vi "SEC code V3.0.1.121.vi"() -> ()   [LabVIEW 2020]
uses:
  SEC code V3.0.1/Drivers and Aux files/IVIUM/IVIUM_remdriver.lvlib
  SEC code V3.0.1/Drivers and Aux files/State.ctl
  SEC code V3.0.1/Drivers and Aux files/SECenumctl.ctl
  SEC code V3.0.1/Drivers and Aux files/OSSPEC.ctl
panel:
  out "?":T1(graph)
  in  "Tab Control 2":T2(tab)
  in  "V 1 time (s)":dbl
  in  "V off time":dbl
  in  "Sampling time (s)":dbl
  in  "V 2 time (s)":dbl
  in  "Run OSPSEC":bool
  out "System potential":dbl
  in  "V1 (V)":dbl
  in  "V2 (V)":dbl
  in  "Reverse Scan\ndirection":bool
  in  "File Name":string="test-1"
  in  "Path":path=path "C:/Users/LocalAdmin/Desktop"
  out "cell on":bool
  in  "Tab Control":T3(tab)
  out "?":T1(graph)
  out "?":T1(graph)
  out "?":cluster{dbl[], dbl[]}(graph)
  out "I_overload":bool
  out "Aninput1_overload":bool
  out "E_overload":bool
  out "cell-off button pressed":bool
  in  "Default\nCurrent range":T4(ring)=enum."100 uA"
  in  "Default Filter":T5(ring)=enum."10 kHz"
  out "Device serial number":string
  in  "Set Stability":T6(ring)=enum."Standard"
  out "Number of Spectrometers":i32
  out "Values to re-intialise to at end\nof the measument":T7
  in  "Equilibration \ntime (s)":u32=5
  in  "Wait before \nspectrum (s)":dbl=0.1
  in  "Inetegration Time (us)":i32=10000
  in  "Continuous \nStrobe Delay (us)":i32
  in  "Increment (V)":dbl=0.01
  in  "Stop potential (V)":dbl=0.4
  in  "Default Potential (V)":dbl=-0.4
  in  "Start potential (V)":dbl=-0.4
  in  "Exit and disconnect":bool
  out "current":dbl caption="Current (A)" format="%_4g"
  out "V (during measurment)":dbl
  out "Potentiostat Status":string
  in  "(update and read)":bool
  # "OSPSEC control"
  # "Program control"
  # "Spectrometer control"
  # "Potentiostat Status"
  # "SEC control"
  # "Cell on?"
  # "I overload overload"
  # "off button pressed"
  # "Aninput1 overload"
  # "E overload"
  # "OSPEC loop exit"
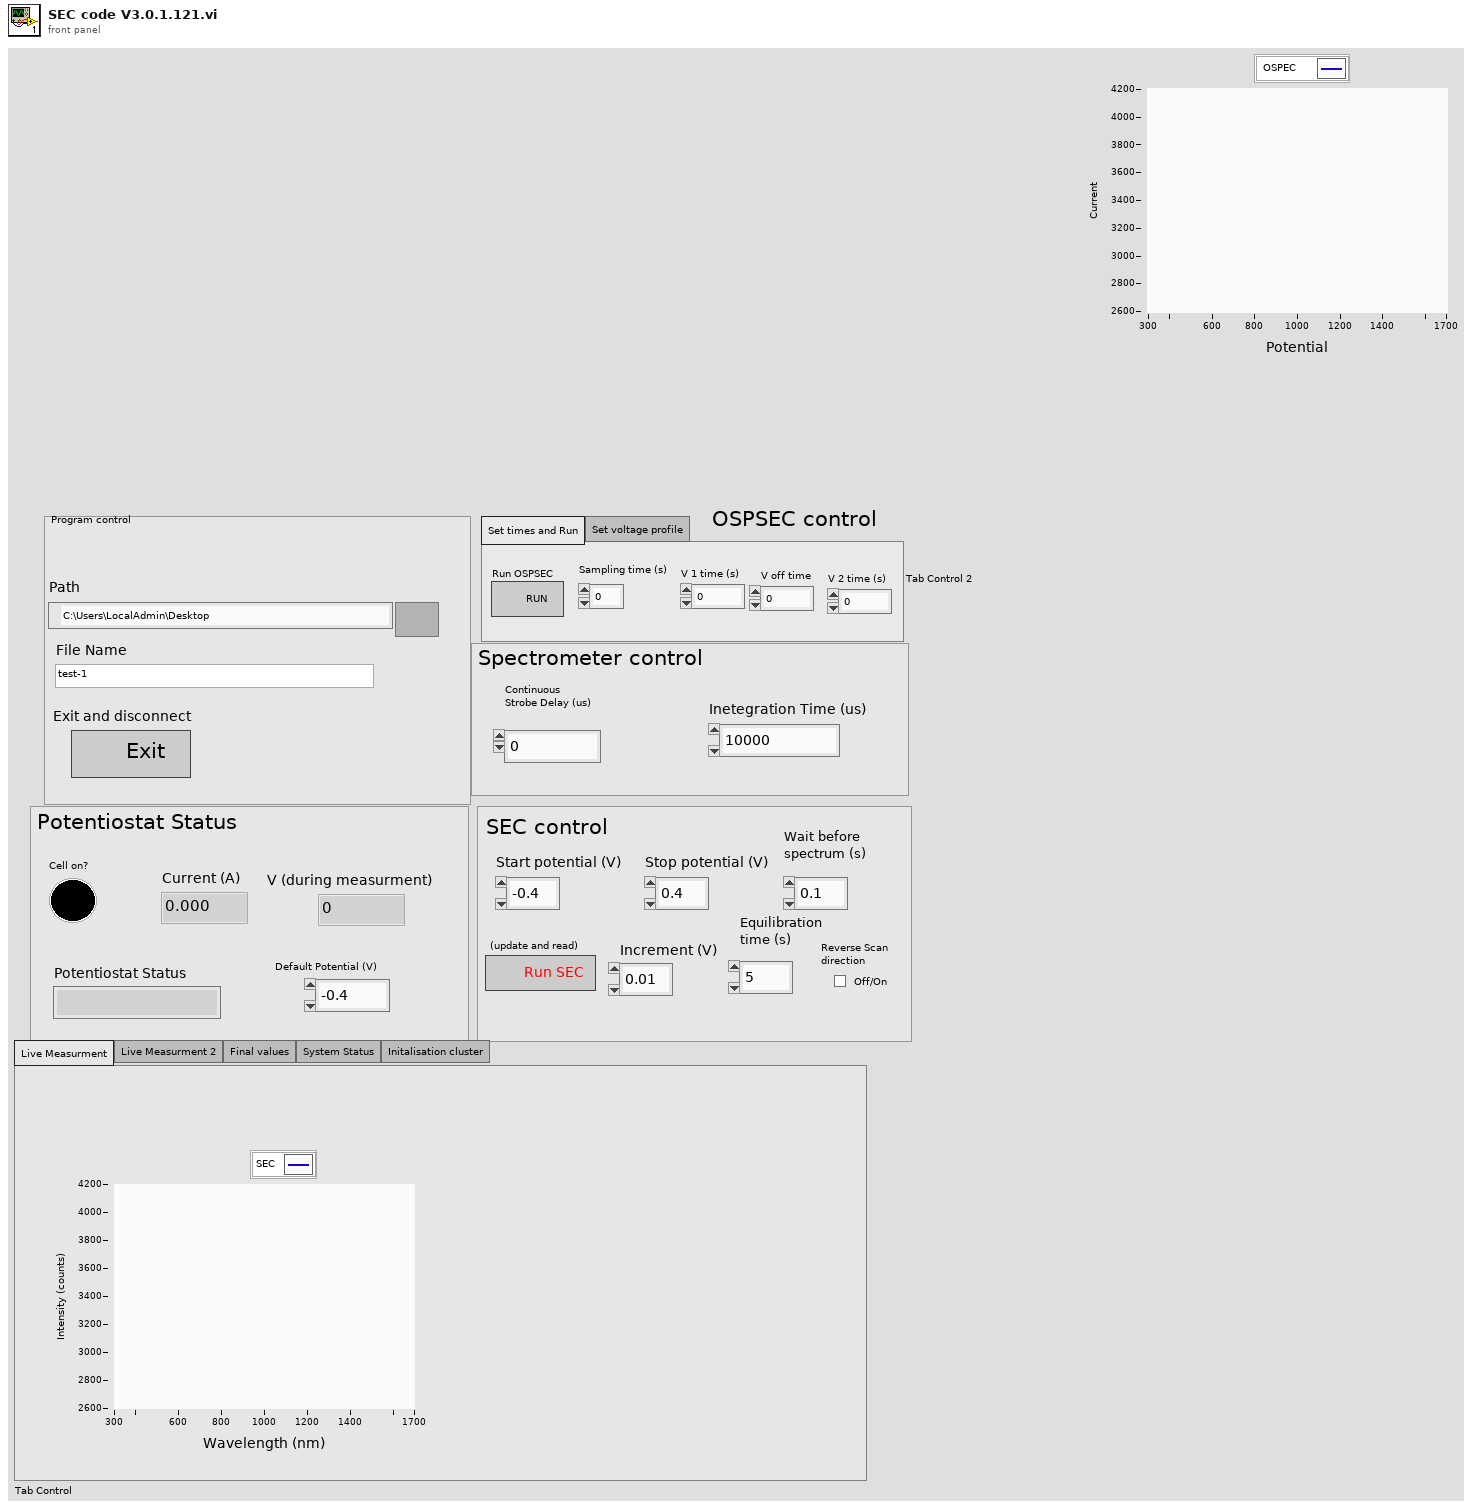
[diagram p1: front panel]
types:
  T1 = cluster{"WL Values":dbl[], "Spectrum Values":dbl[]}
  T2 = enum32{"Set times and Run", "Set voltage profile"}
  T3 = enum32{"Live Measurment", "Live Measurment 2", "Final values", "System Status", "Initalisation cluster"}
  T4 = enum16{"10 A", "1 A", "100 mA", "10 mA", "1 mA", "100 uA", "10 uA", "1 uA", "100 nA", "10 nA", "1 nA", "100 pA", "10 pA", "1 pA"}
  T5 = enum16{"1 MHz", "100 kHz", "10 kHz", "1 kHz", "10 Hz"}
  T6 = enum16{"High Speed", "Standard", "High Stability"}
  T7 = cluster{"Currents":dbl[], "Potentials":dbl[], "Device Status":string, "Device serial no":string, "Current":dbl, "Default \nPotential":dbl, "I overload":bool, "Cell On":bool, "E overload":bool, "Aninput1 overload":bool, "Cell off button pressed":bool, "Start potential":dbl, "Stop potential":dbl, "Increment":dbl, "SEC":dbl[], "Path":path, "File name":string}
  T8 = cluster{"Current array":dbl[], "Potential array":dbl[], "Status":string, "Serial No":string, "Current":dbl, "Default\n potential":dbl, "I overload":bool, "Cell on":bool, "E overload":bool, "Cell of button pressed":bool, "Aninput1 overload":bool, "Stop \npotential":dbl, "Start \npotential":dbl, "Increment":dbl, "Spectrum":dbl[][], "Path":path, "File Name":string, "Sample rate":dbl, "V2 time":dbl, "V off time":dbl, "V 2":dbl, "V 1":dbl, "V1 time":dbl, "Time array":dbl[], "Integration time":i32, "Continous strobe delay":i32, "Time elapsed ":i32, "Start time":i32}
  T9 = typedef "State.ctl" = enum16{"Initialize", "Wait for Event", "Run SEC", "Run OSPEC", "Output data and process", "Exit"}
  T10 = typedef "SECenumctl.ctl" = enum16{"Read spectrum", "Apply potential", "Wait"}
  T11 = typedef "OSSPEC.ctl" = enum16{"Read Potential and spectrum", "Read current and spectrum", "Reinitialise Cell", "Apply V1", "Apply V2"}
  T12 = typedef "Rendezvous RefNum" = refnum<k1>
  T13 = cluster{"Spectrum Values":dbl[], "WL Values":dbl[]}
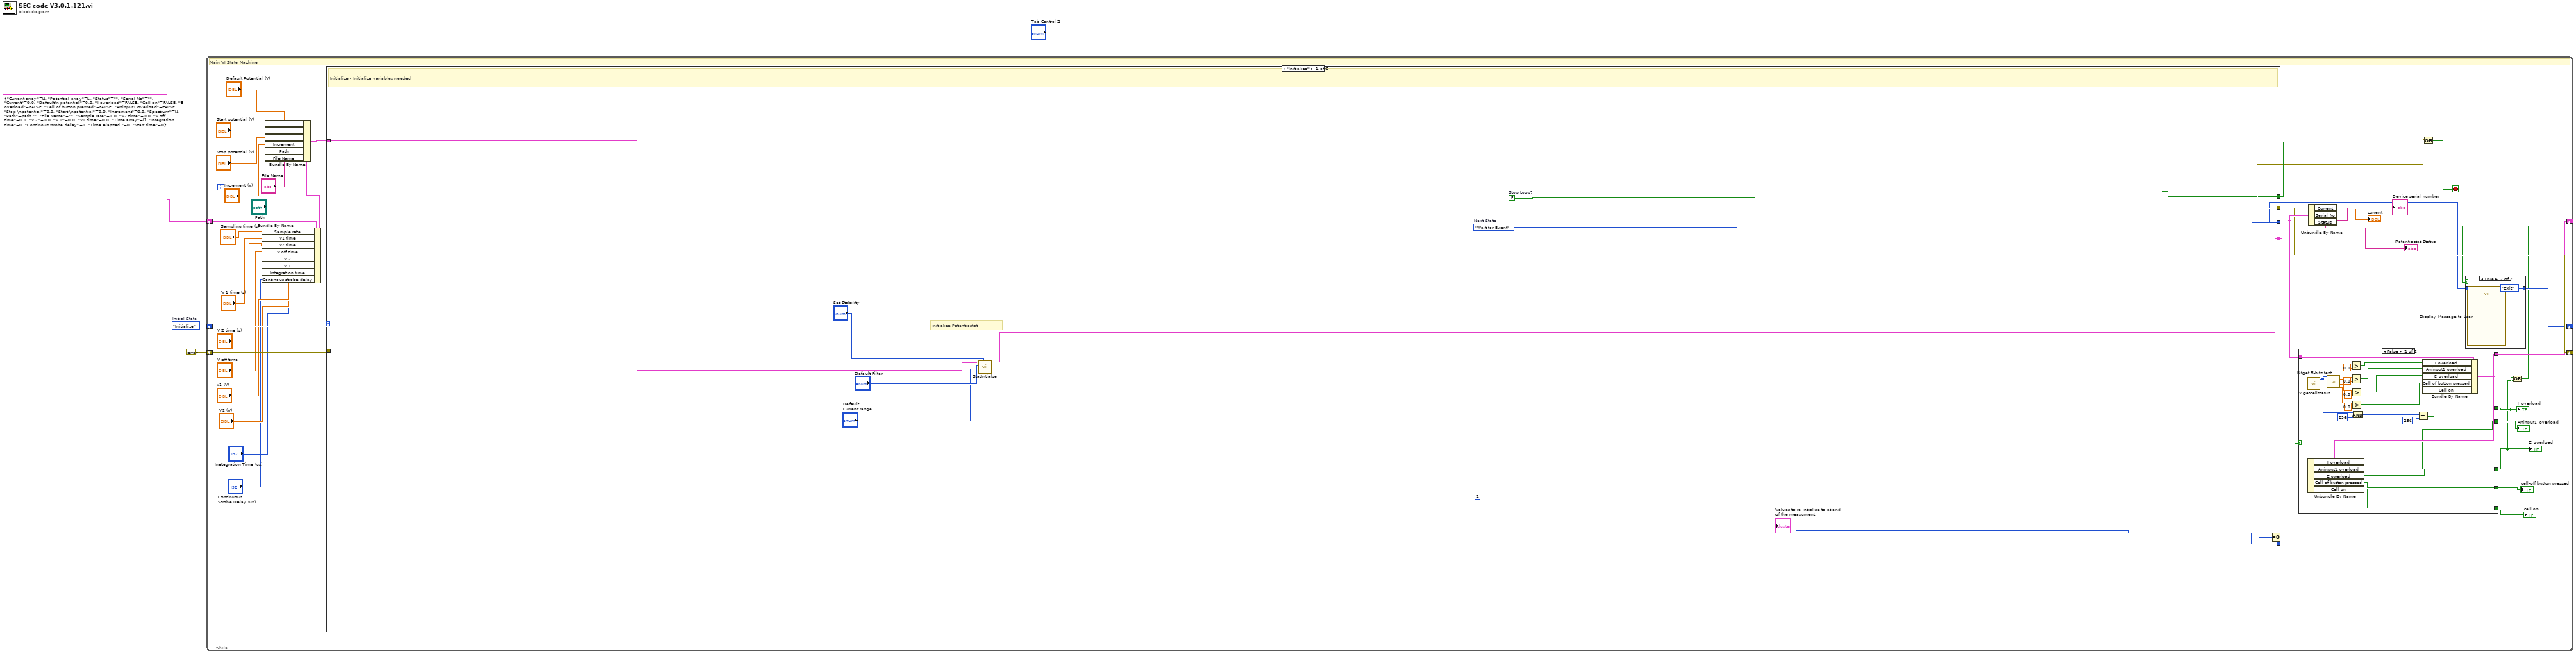
[diagram p0: block diagram]
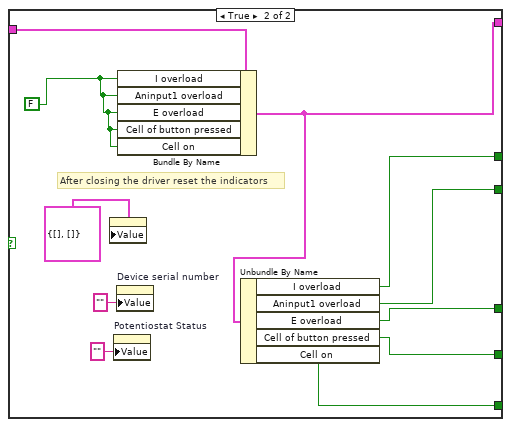
[diagram p3: hidden frame]
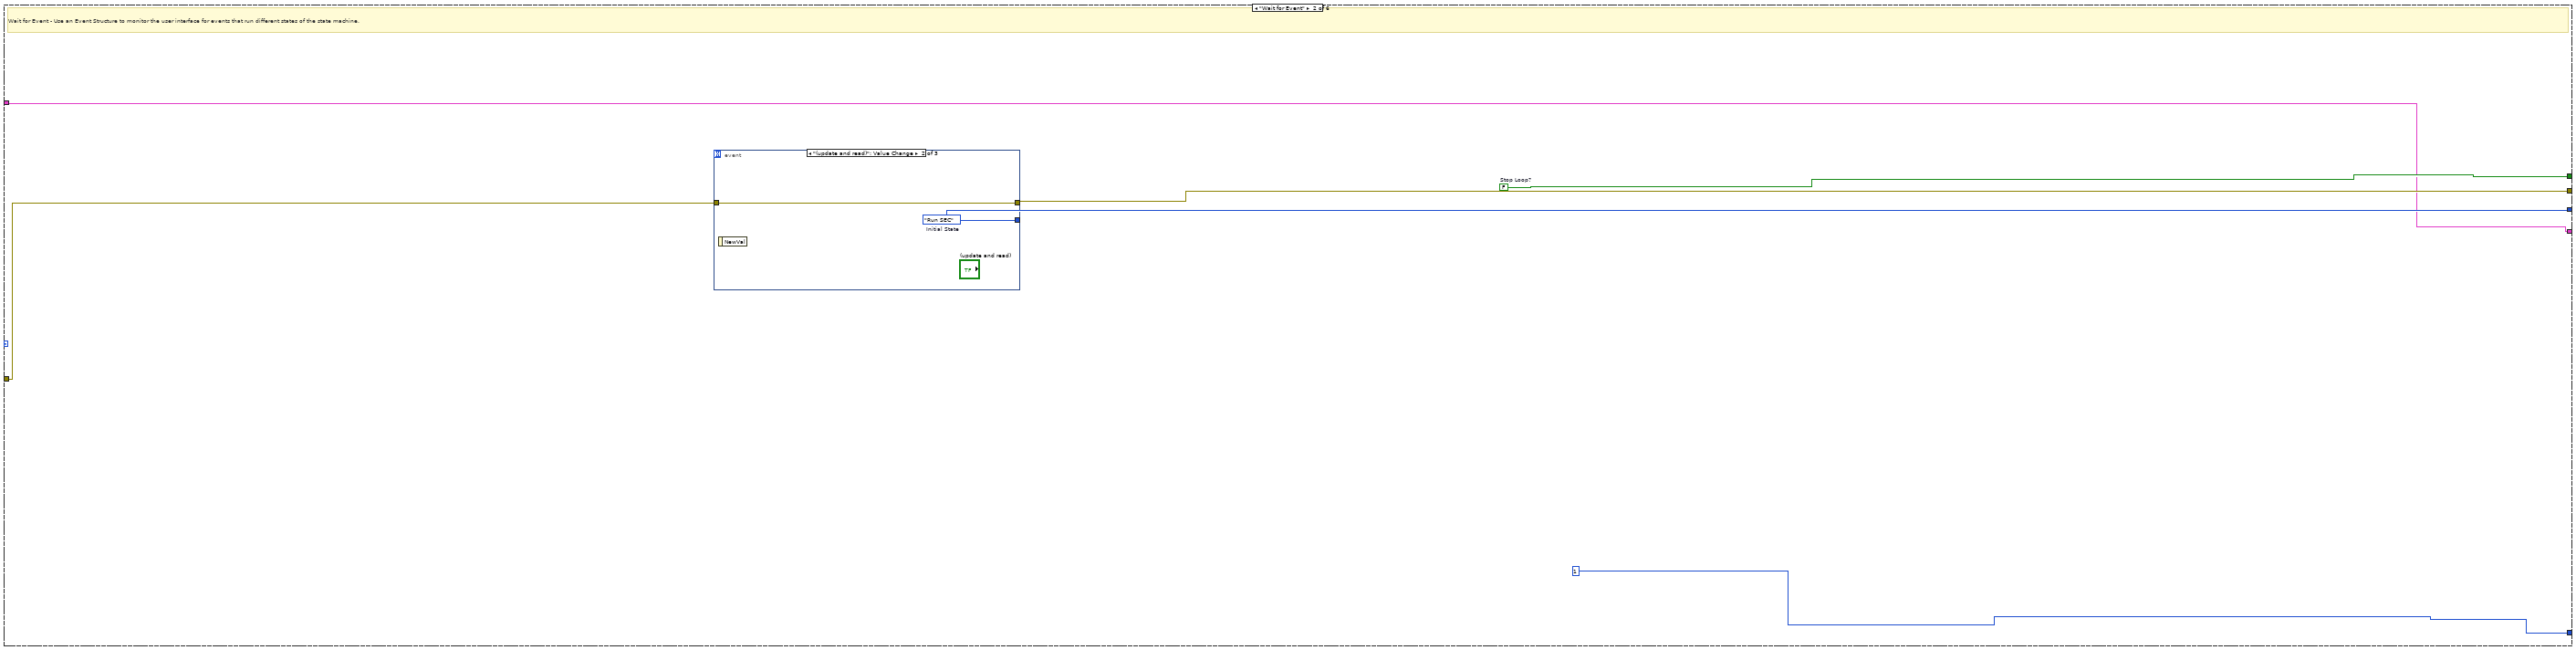
[diagram p4: hidden frame]
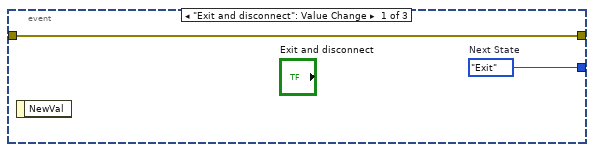
[diagram p5: hidden frame]
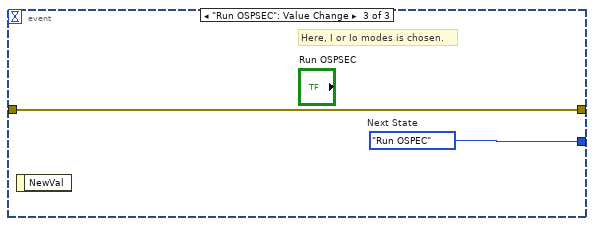
[diagram p6: hidden frame]
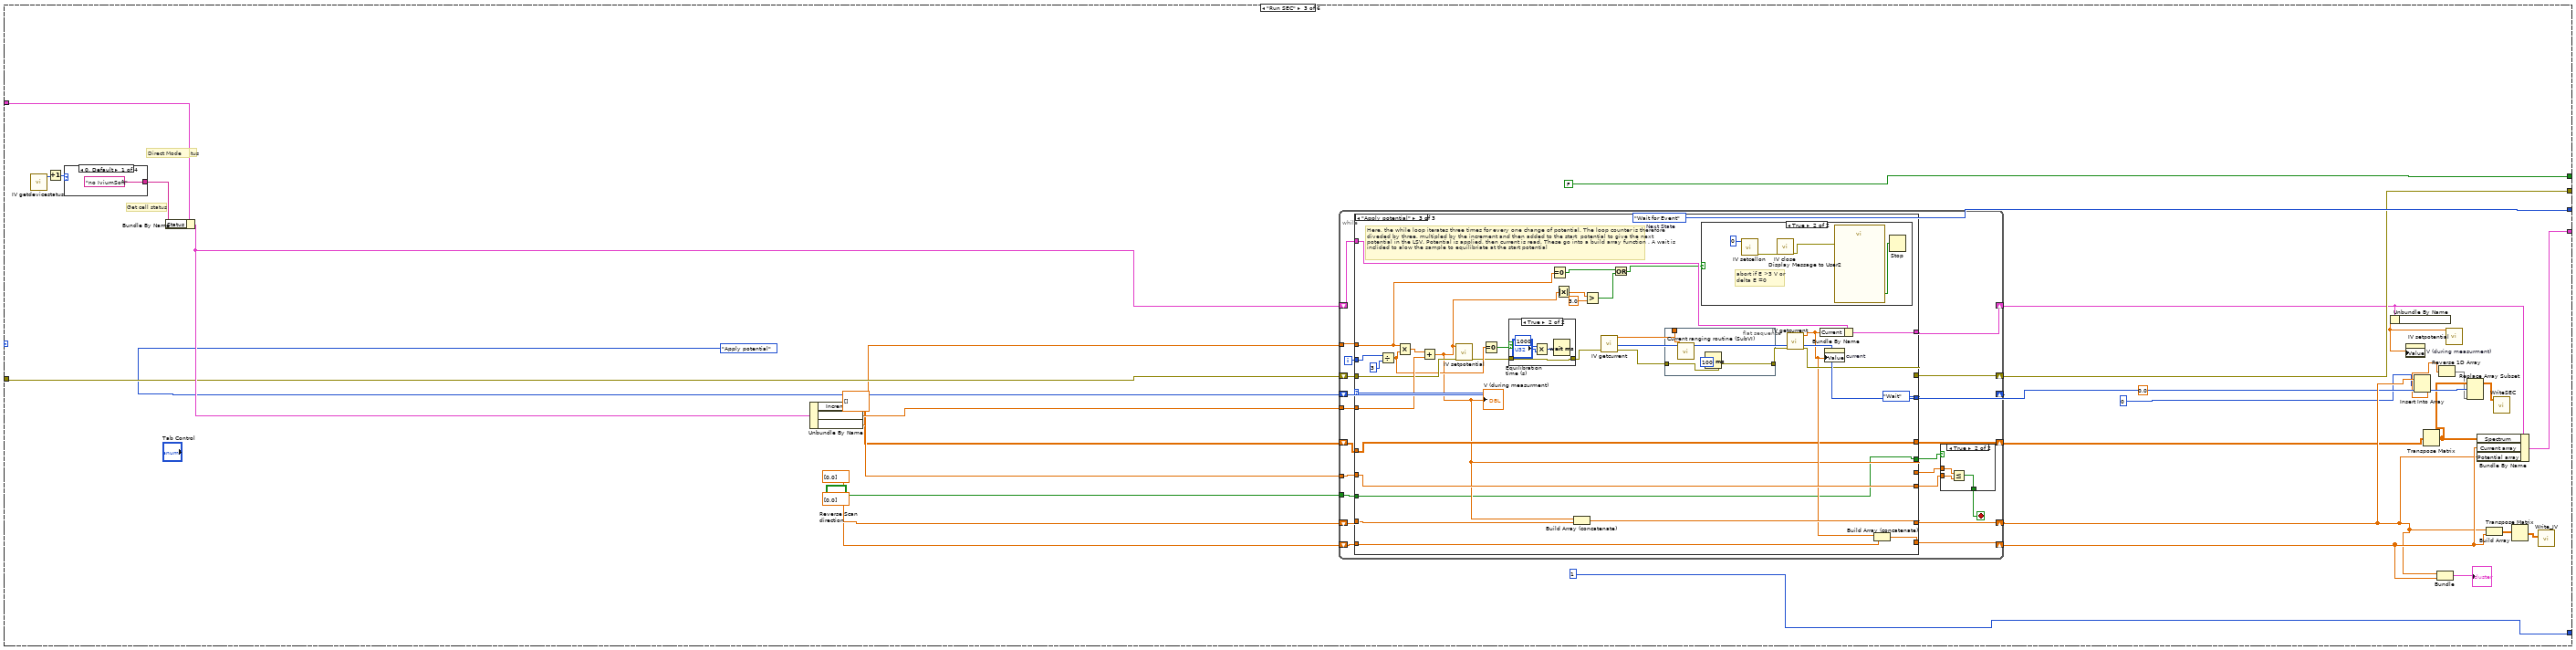
[diagram p7: hidden frame]
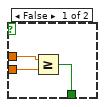
[diagram p8: hidden frame]
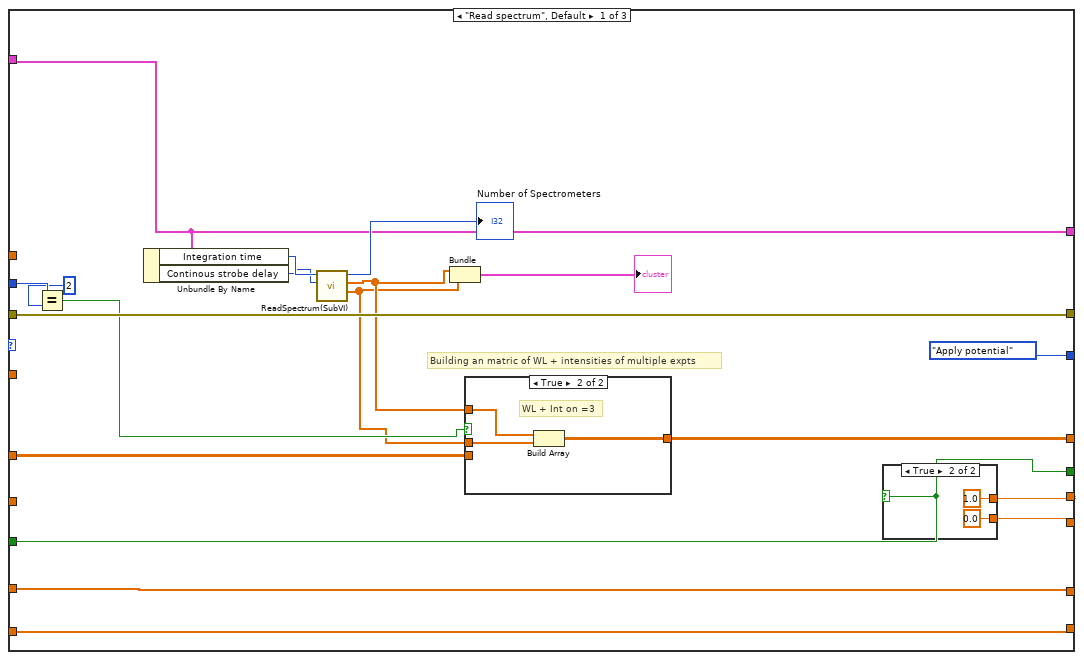
[diagram p9: hidden frame]
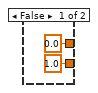
[diagram p10: hidden frame]
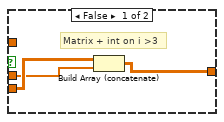
[diagram p11: hidden frame]
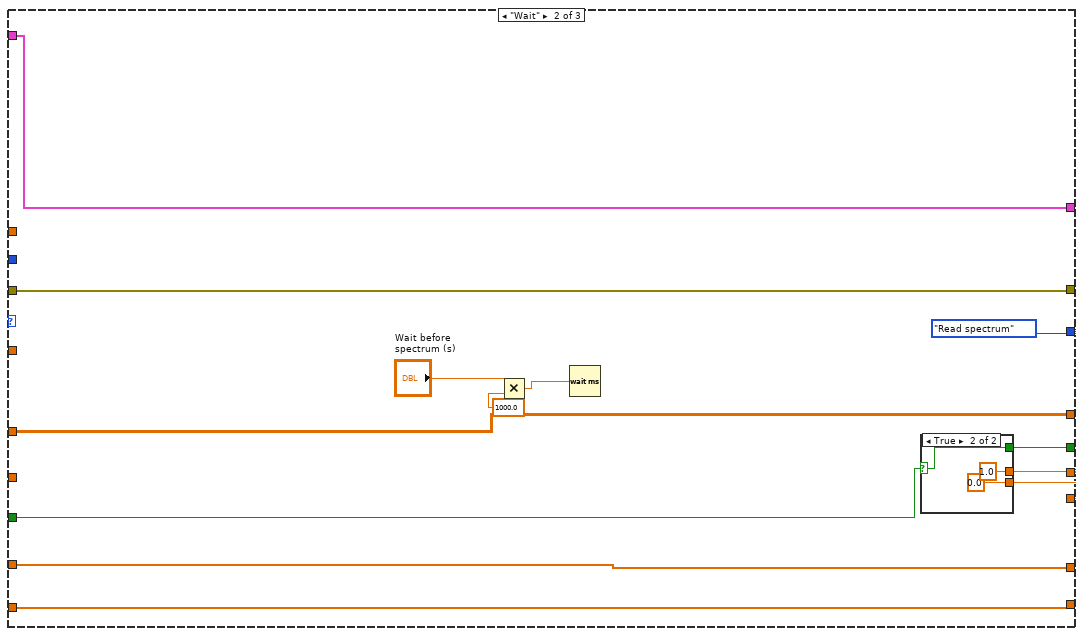
[diagram p12: hidden frame]
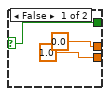
[diagram p13: hidden frame]
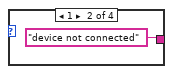
[diagram p16: hidden frame]
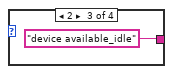
[diagram p17: hidden frame]
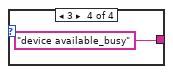
[diagram p18: hidden frame]
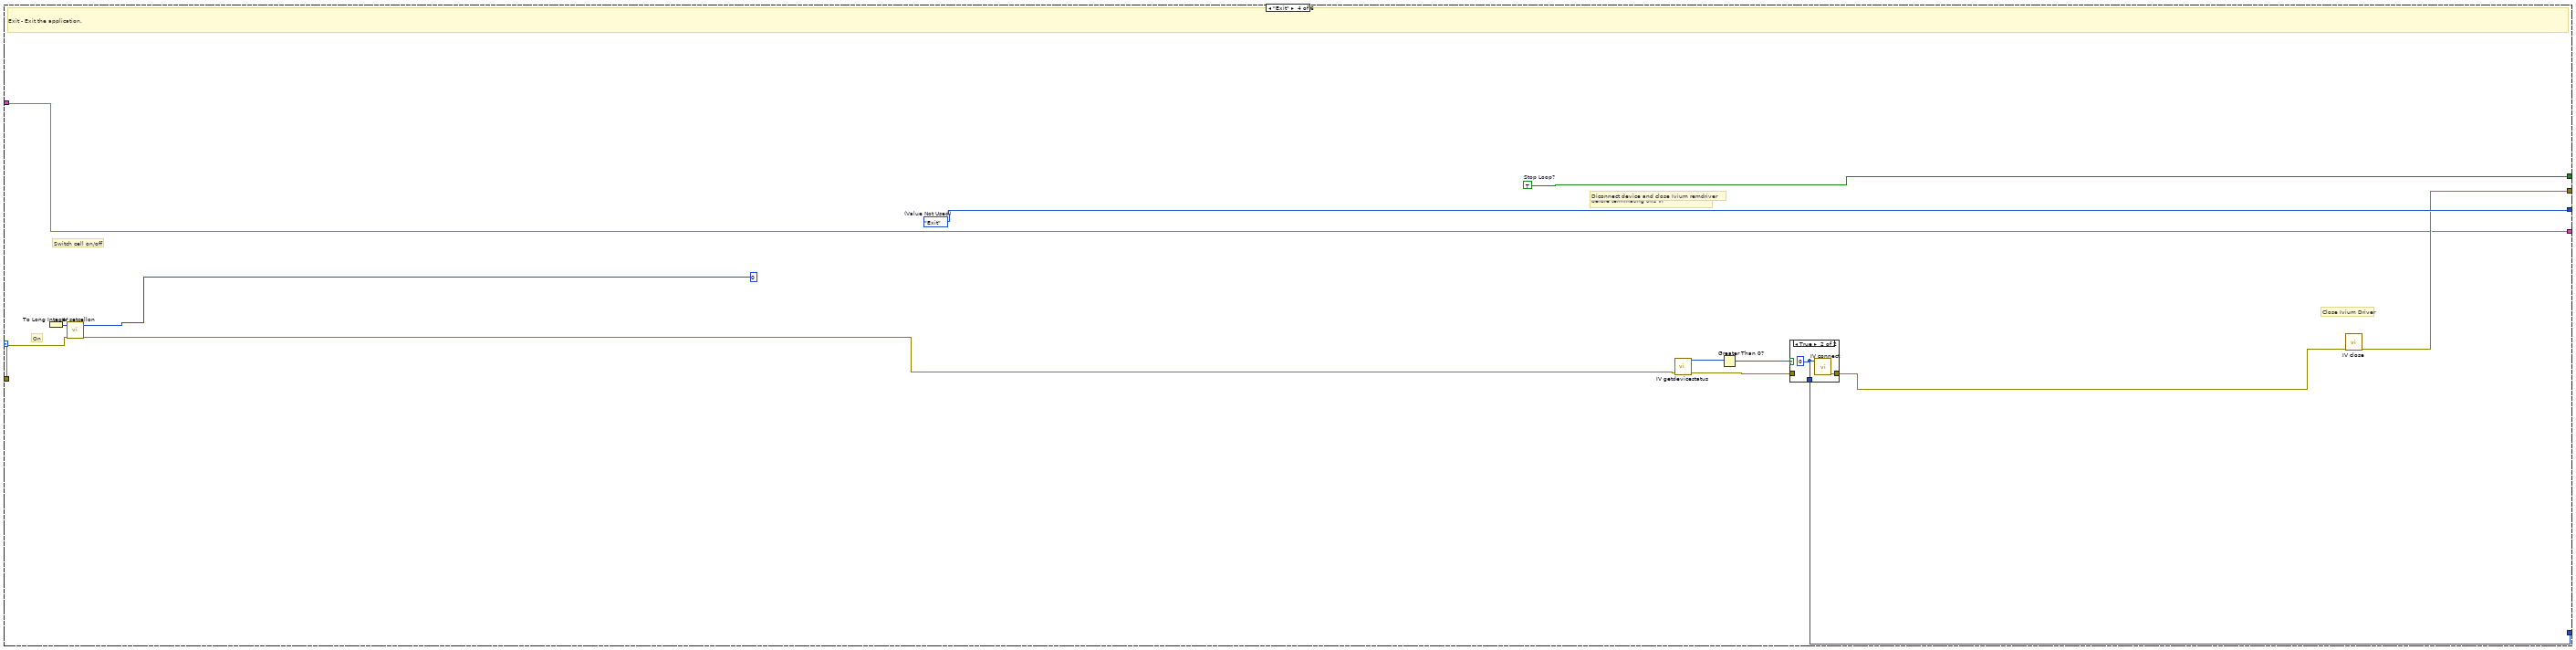
[diagram p19: hidden frame]
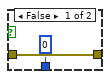
[diagram p20: hidden frame]
diagram:
  w3 = State."Initialize"  # Initial State
  n1 = while {
    shift-right: [w20] -> _
    shift-left: w3 -> [w40]
    shift-right: [w25] -> _
    shift-left: T8 {"Current array"=[], "Potential array"=[], "Status"="", "Serial No"="", "Current"=0.0, "Default\n potential"=0.0, "I overload"=FALSE, "Cell on"=FALSE, "E overload"=FALSE, "Cell of button pressed"=FALSE, "Aninput1 overload"=FALSE, "Stop \npotential"=0.0, "Start \npotential"=0.0, "Increment"=0.0, "Spectrum"=[], "Path"=path "", "File Name"="", "Sample rate"=0.0, "V2 time"=0.0, "V off time"=0.0, "V 2"=0.0, "V 1"=0.0, "V1 time"=0.0, "Time array"=[], "Integration time"=0, "Continous strobe delay"=0, "Time elapsed "=0, "Start time"=0} -> [w13]
    shift-right: [w26] -> _
    shift-left: errorcluster {"status"=FALSE, "code"=0, "source"=""} ("error constant") -> [w39]
    stop <- w37 stop-if-true
    # "Main VI State Machine"
    n2 = Bundle By Name(cluster=w13, "Sample rate"="Sampling time (s)", "V1 time"="V 1 time (s)", "V2 time"="V 2 time (s)", "V off time"="V off time", "V 2"="V1 (V)", "V 1"="V2 (V)", "Integration time"="Inetegration Time (us)", "Continous strobe delay"="Continuous \nStrobe Delay (us)") -> (w4:T8)
    n3 = Bundle By Name(cluster=w4, "Default\n potential"="Default Potential (V)", "Start \npotential"="Start potential (V)", "Stop \npotential"="Stop potential (V)", "Increment"="Increment (V)", "Path"="Path", "File Name"="File Name") -> (w22:T8)
    n4 = case shown="\"Initialize\"" w40 {
      tunnel: [w84 w91 w129 w266 State."Wait for Event" ("f") State."Wait for Event" ("f")] -> w16
      tunnel: [w83 w88 FALSE ("Stop Loop?") w254 FALSE ("Stop Loop?") _] -> w38
      tunnel: w22 -> [w79 w86 w114 w255 w277 w676]
      tunnel: [w78 w86 w104 w255 w272 w676] -> w33
      tunnel: w39 -> [_ w90 w123 w258 w275 w679]
      tunnel: [_ w89 w122 w261 w273 w679] -> w26
      tunnel: [1 ("devconnect") 1 ("devconnect") 1 ("devconnect") w256 1 ("devconnect") 1 ("devconnect")] -> w21
      frame "Initialize" {
        w83 = FALSE  # Stop Loop?
        w84 = State."Wait for Event"  # Next State
        # "initialize Potentiostat"
        # "Initialize - Initialize variables needed"
        n5 = call "StatIntialse.vi"("Set Stability"="Set Stability", "Default\nCurrent range"="Default\nCurrent range", "Default\n Filter"="Default Filter", "Cluster in"=w79) -> ("Cluster out"=w78:T8)  [unwired: 6 in, 1 out]
      }
      frame "Wait for Event" {
        w88 = FALSE  # Stop Loop?
        # "Wait for Event - Use an Event Structure to monitor the user interface for events that run different states of the state machine."
        n6 = event shown="[1] \"(update and read)\": Value Change" {
          selector: _ -> [_ _ _]
          dyn-events: _ -> [_ _ _]
          timeout: _ -> [_ _ _]
          tunnel: [w93 w94 w97] -> w91
          tunnel: w90 -> [w92 w95 w96]
          tunnel: [w92 w95 w96] -> w89
          event "Exit and disconnect": Value Change {
            w93 = State."Exit"  # Next State
            n7 = event-data() -> ()  [unwired: 1 in, 1 out]
          }
          event "(update and read)": Value Change {
            w94 = State."Run SEC"  # Initial State
            n8 = event-data() -> ()  [unwired: 1 in, 1 out]
          }
          event "Run OSPSEC": Value Change {
            w97 = State."Run OSPEC"  # Next State
            # "Here, I or Io modes is chosen."
            n9 = event-data() -> ()  [unwired: 1 in, 1 out]
          }
        }
      }
      frame "Run SEC" {
        w129 = State."Wait for Event"  # Next State
        # "Get cell status"
        # "Get Device Status"
        # "Direct Mode"
        n10 = call "IV getdevicestatus.vi"() -> ("return type"=w127:i32)  [unwired: 10 in, 1 out]
        n11 = Increment(x=w127) -> (x+1=w126:i32)
        n12 = case shown="0, Default" w126 {
          tunnel: ["no IviumSoft" "device not connected" "device available_idle" "device available_busy"] -> w131
          frame 0, Default {
          }
          frame 1 {
          }
          frame 2 {
          }
          frame 3 {
          }
        }
        n13 = Bundle By Name(cluster=w114, "Status"=w131) -> (w125:T8)
        n14 = Unbundle By Name(w125) -> ("Increment"=w120:dbl, "Start \npotential"=w124:dbl, "Stop \npotential"=w115:dbl)
        n15 = while {
          shift-right: [w151] -> w106
          shift-left: w125 -> [w152]
          tunnel: w120 -> [w147]
          tunnel: w124 -> [w146]
          shift-right: [w148] -> w122
          shift-left: w123 -> [w149]
          shift-right: [w140] -> _
          shift-left: SECenumctl."Apply potential" -> [w144]
          shift-right: [w142] -> w111
          shift-left: dbl[] [0.0] -> [w141]
          shift-right: [w137] -> w112
          shift-left: dbl[] [0.0] -> [w138]
          tunnel: w115 -> [w139]
          shift-right: [w136] -> w110
          shift-left: dbl[][] [] -> [w135]
          tunnel: "Reverse Scan\ndirection" -> [w133]
          i -> [w150]
          stop <- w134 stop-if-true
          n16 = case shown="\"Apply potential\"" w144 {
            tunnel: w152 -> [w161 w199 w221]
            tunnel: [w161 w199 w220] -> w151
            tunnel: w150 -> [w170 _ w235]
            tunnel: w149 -> [w171 w195 w232]
            tunnel: [w171 w195 w222] -> w148
            tunnel: w147 -> [_ _ w217]
            tunnel: w146 -> [_ _ w234]
            tunnel: [w177 w198 w214] -> w145
            tunnel: [w176 w197 w227] -> w143
            tunnel: [w175 w196 w225] -> w142
            tunnel: w141 -> [w175 w196 w226]
            tunnel: [SECenumctl."Apply potential" SECenumctl."Read spectrum" SECenumctl."Wait"] -> w140
            tunnel: w139 -> [_ _ w227]
            tunnel: w138 -> [w172 w191 w224]
            tunnel: [w172 w191 w223] -> w137
            tunnel: [w164 w190 w218] -> w136
            tunnel: w135 -> [w163 w190 w218]
            tunnel: w133 -> [w162 w189 w207]
            tunnel: [w162 w188 w207] -> w132
            frame "Read spectrum", Default {
              # "Building an matric of WL + intensities of multiple expts"
              n17 = Equal?(x=w170, y=2) -> (x = y?=w168:bool)
              n18 = Unbundle By Name(w161) -> ("Integration time"=w160:i32, "Continous strobe delay"=w159:i32)
              n19 = call "ReadSpectrum(SubVI).vi"("Continuous \nStrobe Delay"=w159, "Enter the \nInetegration Time"=w160) -> ("Spectrum Values"=w166:dbl[], "WL Values"=w167:dbl[], "Number of Spectrometers"=→"Number of Spectrometers":i32)  [unwired: 7 in]
              n20 = Bundle("WL Values"=w167, "Spectrum Values"=w166) -> (→"?":T1)  [unwired: 1 in]
              n21 = case shown="True" w168 {
                tunnel: w167 -> [_ w187]
                tunnel: w166 -> [w183 w186]
                tunnel: [w182 w185] -> w164
                tunnel: w163 -> [w184 _]
                frame False {
                  # "Matrix + int on i >3"
                  n22 = Build Array (concatenate)(w184, w183) -> (w182:dbl[][])
                }
                frame True {
                  # "WL + Int on =3"
                  n23 = Build Array(w187, w186) -> (w185:dbl[][])
                }
              }
              n24 = case shown="True" w162 {
                tunnel: [0.0 1.0] -> w177
                tunnel: [1.0 ("Stop \npotential") 0.0 ("Stop \npotential")] -> w176
                frame False {
                }
                frame True {
                }
              }
            }
            frame "Wait" {
              n25 = Multiply(x="Wait before \nspectrum (s)", y=1000.0) -> (x*y=w194:dbl)
              n26 = Wait (ms)(milliseconds to wait=w194) -> ()  [unwired: 1 out]
              n27 = case shown="True" w189 {
                selector: w189 -> [w201 w204]
                tunnel: [0.0 1.0] -> w198
                tunnel: [1.0 ("Stop \npotential") 0.0 ("Stop \npotential")] -> w197
                tunnel: [w201 w204] -> w188
                frame False {
                }
                frame True {
                }
              }
            }
            frame "Apply potential" {
              # "Here, the while loop iterates three times for every one change of potential. The loop counter is therefore diveded by three, multipled by the increment and then added to the start  potential to give the next potential in the LSV. Potential is applied, then current is read. These go into a build array function . A wait is inclided to alow the sample to equilibriate at the start potential"
              n28 = Divide(x=w235, y=3) -> (x/y=w230:dbl)
              n29 = Multiply(x=w217, y=w230) -> (x*y=w233:dbl)
              n30 = Add(x=w233, y=w234) -> (x+y=w214:dbl)
              "V (during measurment)" <- w214
              n31 = call "IV setpotential.vi"("error in (no error)"=w232, "value"=w214) -> ("error out"=w229:errorcluster)  [unwired: 7 in, 2 out]
              n32 = Equal To 0?(x=w230) -> (x = 0?=w231:bool)
              n33 = case shown="True" w231 {
                tunnel: w229 -> [w245 w247]
                tunnel: [w245 w247] -> w228
                frame False {
                }
                frame True {
                  n34 = Multiply(x=u32 1000, y="Equilibration \ntime (s)") -> (x*y=w246:u32)
                  n35 = Wait (ms)(milliseconds to wait=w246) -> ()  [unwired: 1 out]
                }
              }
              n36 = Equal To 0?(x=w217) -> (x = 0?=w212:bool)
              n37 = Absolute Value(x=w214) -> (abs(x)=w215:dbl)
              n38 = Build Array (concatenate)(w214, w226) -> (w225:dbl[])
              n39 = Greater?(x=w215, y=3.0) -> (0:w213:bool)
              n40 = call "IV getcurrent.vi"("error in (no error)"=w228) -> ("error out"=w210:errorcluster, "value out"=w208:dbl)  [unwired: 8 in, 1 out]
              n41 = Or(x=w212, y=w213) -> (x .or. y?=w211:bool)
              n42 = flat-sequence {
                tunnel: w210 -> [w239]
                tunnel: [w239] -> w209
                tunnel: w208 -> [w238]
                frame #0 {
                  n43 = call "Current ranging routine (SubVI).vi"("Current"=w238) -> ()  [unwired: 11 in]
                  n44 = Wait (ms)(milliseconds to wait=u32 100) -> ()  [unwired: 1 out]
                }
              }
              n45 = case shown="True" w211 {
                frame False {
                }
                frame True {
                  # "abort if E >3 V or\ndelta E =0"
                  n46 = call "IV setcellon.vi"("cellon"=0) -> ("error out"=w243:errorcluster)  [unwired: 8 in, 2 out]
                  n47 = call "IV close.vi"("error in (no error)"=w243) -> ("error out"=w241:errorcluster)  [unwired: 9 in, 1 out]
                  n48 = call "Display Message to User2"("error in (no error)"=w241) -> ("OK"=w244:bool)  [unwired: 9 in, 1 out]
                  n49 = Stop(stop? (T)=w244) -> ()
                }
              }
              n50 = call "IV getcurrent.vi"("error in (no error)"=w209) -> ("error out"=w222:errorcluster, "value out"=w219:dbl)  [unwired: 8 in, 1 out]
              n51 = Bundle By Name(cluster=w221, "Current"=w219) -> (w220:T8)
              n52 = property on="current" class="DigNum (strict)"("Value"=w219) -> ()  [unwired: 2 in, 2 out]
              n53 = Build Array (concatenate)(w219, w224) -> (w223:dbl[])
            }
          }
          n54 = case shown="True" w132 {
            tunnel: w145 -> [w155 w157]
            tunnel: w143 -> [w154 w156]
            tunnel: [w153 w158] -> w134
            frame False {
              n55 = Greater Or Equal?(x=w155, y=w154) -> (x >= y?=w153:bool)
            }
            frame True {
              n56 = Less Or Equal?(x=w157, y=w156) -> (x <= y?=w158:bool)
            }
          }
        }
        n57 = Unbundle By Name(w106) -> ("Default\n potential"=w119:dbl)
        n58 = property on="V (during measurment)" class="DigNum (strict)"("Value"=w119) -> ()  [unwired: 2 in, 2 out]
        n59 = Insert Into Array(array=w111, index=0, new element=0.0 ("new element/subarray")) -> (w102:dbl[])
        n60 = Transpose Matrix(1:w110) -> (0:w108:dbl[][])
        n61 = Bundle(w111, w112) -> (→"?":cluster{dbl[], dbl[]})  [unwired: 1 in]
        n62 = Reverse 1D Array(array=w102) -> (reversed array=w101:dbl[])
        n63 = call "IV setpotential.vi"("value"=w119) -> ()  [unwired: 8 in, 3 out]
        n64 = Replace Array Subset(array=w108, new element=w101, index (row)=0 ("index")) -> (w107:dbl[][])  [unwired: 1 in]
        n65 = Bundle By Name(cluster=w106, "Spectrum"=w108, "Current array"=w112, "Potential array"=w111) -> (w104:T8)
        n66 = Build Array(w111, w112) -> (w105:dbl[][])
        n67 = call "WriteSEC.vi"("Array"=w107) -> ()  [unwired: 11 in]
        n68 = Transpose Matrix(1:w105) -> (0:w103:dbl[][])
        n69 = call "Write_JV.vi"("Array"=w103) -> ()  [unwired: 11 in]
      }
      frame "Exit" {
        w254 = TRUE  # Stop Loop?
        w266 = State."Exit"  # (Value Not Used)
        # "On"
        # "Switch cell on/off"
        # "Diconnect device and close Ivium remdriver"
        # "Disconnect Ivium device (when connected)\nbefore terminating this VI"
        # "Close Ivium Driver"
        # "Exit - Exit the application."
        n70 = To Long Integer(number=0) -> (32bit integer=w260:i32)
        n71 = call "IV setcellon.vi"("error in (no error)"=w258, "cellon"=w260) -> ("error out"=w257:errorcluster)  [unwired: 7 in, 2 out]
        n72 = call "IV getdevicestatus.vi"("error in (no error)"=w257) -> ("error out"=w262:errorcluster, "return type"=w264:i32)  [unwired: 9 in]
        n73 = Greater Than 0?(x=w264) -> (x > 0?=w263:bool)
        n74 = case shown="True" w263 {
          tunnel: [w268 w270] -> w265
          tunnel: w262 -> [w268 _]
          tunnel: [0 ("devconnect") w269] -> w256
          frame False {
          }
          frame True {
            w269 = 0 ("devconnect")
            n75 = call "IV connect.vi"("devconnect"=w269) -> ("error out"=w270:errorcluster)  [unwired: 8 in, 2 out]
          }
        }
        n76 = call "IV close.vi"("error in (no error)"=w265) -> ("error out"=w261:errorcluster)  [unwired: 9 in, 1 out]
      }
      frame "Run OSPEC" {
        # "Get cell status"
        # "Get Device Status"
        # "Direct Mode"
        n77 = call "IV getdevicestatus.vi"() -> ("return type"=w280:i32)  [unwired: 10 in, 1 out]
        n78 = Increment(x=w280) -> (x+1=w279:i32)
        n79 = case shown="0, Default" w279 {
          tunnel: ["no IviumSoft" "device not connected" "device available_idle" "device available_busy"] -> w278
          frame 0, Default {
          }
          frame 1 {
          }
          frame 2 {
          }
          frame 3 {
          }
        }
        n80 = Bundle By Name(cluster=w277, "Status"=w278) -> (w276:T8)
        n81 = while {
          shift-right: [w290] -> w273
          shift-left: w275 -> [w292]
          shift-right: [w285] -> w272
          shift-left: w276 -> [w294]
          shift-right: [w291] -> _
          shift-left: OSSPEC."Apply V1" -> [w293]
          i -> [w289]
          stop <- w283 stop-if-true
          n82 = case shown="\"Apply V2\"" w293 {
            tunnel: w294 -> [w306 w422 w582 w613 w644]
            tunnel: w292 -> [w302 w417 w588 w607 w647]
            tunnel: [_ w424 OSSPEC."Read Potential and spectrum" OSSPEC."Read current and spectrum" OSSPEC."Read current and spectrum"] -> w291
            tunnel: [w300 w419 w585 w608 w648] -> w290
            tunnel: [w297 w425 w582 w604 w644] -> w288
            tunnel: w289 -> [_ w427 _ _ _]
            tunnel: [w303 w423 w581 w603 w643] -> w287
            tunnel: [w296 w420 w580 w602 w642] -> w286
            tunnel: [w298 _ w579 w601 w641] -> w284
            tunnel: [TRUE FALSE FALSE FALSE FALSE] -> w283
            frame "Read Potential and spectrum", Default {
              n83 = call <vilib>:"Create Rendezvous.vi"("size (2)"=3) -> ("rendezvous"=w309:T12)  [unwired: 4 in, 2 out]
              n84 = Obtain Notifier(name (unnamed)="Stop loops", notification data type=FALSE) -> (notifier out=w308:refnum<notifier>)  [unwired: 2 in, 2 out]
              n85 = Unbundle By Name(w306) -> ("Integration time"=w312:i32, "Continous strobe delay"=w311:i32, "Sample rate"=w310:dbl, "Potential array"=w305:dbl[], "Spectrum"=w304:dbl[][])
              n86 = while {
                tunnel: [w407] -> w307
                shift-right: [w401] -> w297
                shift-left: w306 -> [w404]
                tunnel: w309 -> [w398]
                tunnel: w308 -> [w397]
                stop <- w408 stop-if-true
                n87 = flat-sequence {
                  tunnel: w398 -> [w409]
                  tunnel: w404 -> [w414]
                  tunnel: [w412] -> w403
                  frame #0 {
                    n88 = call <vilib>:"Wait at Rendezvous.vi"("rendezvous"=w409) -> ()  [unwired: 4 in, 3 out]
                  }
                  frame #1 {
                    n89 = Unbundle By Name(w414) -> ("Start time"=w410:i32)
                    n90 = Tick Count (ms)() -> (millisecond timer value=w411:u32)
                    n91 = Subtract(x=w411, y=w410) -> (x-y=w413:u32)
                    n92 = Bundle By Name(cluster=w414, "Time elapsed"=w413) -> (w412:T8)
                  }
                }
                n93 = Unbundle By Name(w403) -> ("Time elapsed"=w400:i32, "V off time"=w399:dbl)
                n94 = Unbundle By Name(w403) -> ("Time array"=w406:dbl[])
                n95 = Greater Or Equal?(x=w400, y=w399) -> (x >= y?=w408:bool)
                n96 = Coerce To Type(0:w400, 1:w399) -> (2:w405:dbl)
                n97 = Send Notification(notification=w408, notifier=w397) -> (notifier out=w407:refnum<notifier>)  [unwired: 1 in, 1 out]
                n98 = Build Array (concatenate)(w406, w405) -> (w402:dbl[])
                n99 = Bundle By Name(cluster=w403, "Time array"=w402) -> (w401:T8)
              }
              n100 = while {
                tunnel: w309 -> [w362]
                tunnel: [w361] -> w301
                tunnel: w308 -> [w357]
                tunnel: w312 -> [w352]
                tunnel: w311 -> [w349]
                tunnel: w310 -> [w348]
                shift-right: [w345] -> w303
                shift-left: w304 -> [w341]
                tunnel: w302 -> [w339]
                stop <- w355 stop-if-true
                n101 = flat-sequence {
                  tunnel: [w372] -> w363
                  tunnel: w362 -> [w372]
                  tunnel: [w371] -> w358
                  tunnel: w357 -> [w371]
                  tunnel: [w370] -> w353
                  tunnel: w352 -> [w370]
                  tunnel: [w369] -> w350
                  tunnel: w349 -> [w369]
                  tunnel: w348 -> [w368]
                  tunnel: [w367] -> w342
                  tunnel: w341 -> [w367]
                  tunnel: [w366] -> w340
                  tunnel: w339 -> [w366]
                  tunnel: [w381] -> w365
                  tunnel: w363 -> [w380]
                  tunnel: [w379] -> w359
                  tunnel: w358 -> [w379]
                  tunnel: [w378] -> w354
                  tunnel: w353 -> [w378]
                  tunnel: [w377] -> w351
                  tunnel: w350 -> [w377]
                  tunnel: [w376] -> w343
                  tunnel: w342 -> [w376]
                  tunnel: w340 -> [w375]
                  tunnel: w365 -> [w389]
                  tunnel: [w389] -> w364
                  tunnel: [w388] -> w360
                  tunnel: w359 -> [w388]
                  tunnel: w354 -> [w387]
                  tunnel: w351 -> [w386]
                  tunnel: [w385] -> w347
                  tunnel: [w384] -> w346
                  tunnel: [w383] -> w344
                  tunnel: w343 -> [w383]
                  tunnel: [w396] -> w361
                  tunnel: w364 -> [w396]
                  tunnel: [w395] -> w356
                  tunnel: w360 -> [w395]
                  tunnel: w347 -> [w391]
                  tunnel: w346 -> [w390]
                  tunnel: [w394] -> w345
                  tunnel: w344 -> [w393]
                  frame #0 {
                    n102 = Multiply(x=w368, y=1000.0) -> (x*y=w374:dbl)
                    n103 = Wait (ms)(milliseconds to wait=w374) -> ()  [unwired: 1 out]
                  }
                  frame #1 {
                    n104 = call <vilib>:"Wait at Rendezvous.vi"("error in (no error)"=w375, "rendezvous"=w380) -> ("error out"=w381:errorcluster)  [unwired: 3 in, 2 out]
                  }
                  frame #2 {
                    n105 = call "ReadSpectrum(SubVI).vi"("Continuous \nStrobe Delay"=w386, "Enter the \nInetegration Time"=w387) -> ("Spectrum Values"=w384:dbl[], "WL Values"=w385:dbl[], "Number of Spectrometers"=w382:i32)  [unwired: 7 in]
                    n106 = property on="Number of Spectrometers" class="DigNum (strict)"("Value"=w382) -> ()  [unwired: 2 in, 2 out]
                  }
                  frame #3 {
                    n107 = Build Array (concatenate)(w393, w391) -> (w394:dbl[][])
                    n108 = Bundle("Spectrum Values"=w390, "WL Values"=w391) -> (→"?":T13)  [unwired: 1 in]
                  }
                }
                n109 = Wait on Notification(notifier=w356) -> (notification=w355:bool)  [unwired: 3 in, 3 out]
              }
              n110 = while {
                shift-right: [w327] -> w299
                shift-left: _ -> [w316]
                tunnel: w309 -> [w326]
                tunnel: w308 -> [w324]
                shift-right: [w321] -> w298
                shift-left: w305 -> [w317]
                stop <- w322 stop-if-true
                n111 = flat-sequence {
                  tunnel: [w333] -> w328
                  tunnel: [w331] -> w325
                  tunnel: [w330] -> w318
                  tunnel: w326 -> [w332]
                  tunnel: w324 -> [w331]
                  tunnel: w317 -> [w330]
                  tunnel: w316 -> [w329]
                  tunnel: [w335] -> w327
                  tunnel: [w334] -> w320
                  tunnel: w328 -> [w336]
                  tunnel: [w338] -> w323
                  tunnel: w325 -> [w338]
                  tunnel: [w337] -> w319
                  tunnel: w318 -> [w337]
                  frame #0 {
                    n112 = call <vilib>:"Wait at Rendezvous.vi"("error in (no error)"=w329, "rendezvous"=w332) -> ("error out"=w333:errorcluster)  [unwired: 3 in, 2 out]
                  }
                  frame #1 {
                    # "Building a 1d matrix of potentials"
                    n113 = call "IV getpotential.vi"("error in (no error)"=w336) -> ("error out"=w335:errorcluster, "value out"=w334:dbl)  [unwired: 8 in, 1 out]
                  }
                }
                n114 = Wait on Notification(notifier=w323) -> (notification=w322:bool)  [unwired: 3 in, 3 out]
                n115 = Build Array (concatenate)(w319, w320) -> (w321:dbl[])
              }
              n116 = Release Notifier(notifier=w307) -> ()  [unwired: 2 in, 3 out]
              n117 = Unbundle By Name(w297) -> ("Current array"=w296:dbl[])
              n118 = Merge Errors(w301, w299) -> (w300:errorcluster)
            }
            frame "Read current and spectrum" {
              n119 = Unbundle By Name(w422) -> ("Integration time"=w430:i32, "Continous strobe delay"=w429:i32, "Sample rate"=w428:dbl)
              n120 = call <vilib>:"Create Rendezvous.vi"("size (2)"=3) -> ("rendezvous"=w435:T12)  [unwired: 4 in, 2 out]
              n121 = Obtain Notifier(name (unnamed)="Stop loops", notification data type=FALSE) -> (notifier out=w431:refnum<notifier>)  [unwired: 2 in, 2 out]
              n122 = Unbundle By Name(w422) -> ("Current array"=w421:dbl[])
              n123 = while {
                tunnel: w435 -> [w497]
                tunnel: w431 -> [w492]
                tunnel: w430 -> [w487]
                tunnel: w429 -> [w484]
                tunnel: w428 -> [w483]
                tunnel: w427 -> [w479]
                shift-right: [w476] -> w423
                shift-left: _ -> [w472]
                shift-right: [w496] -> w416
                shift-left: w417 -> [_]
                stop <- w490 stop-if-true
                n124 = flat-sequence {
                  tunnel: [w507] -> w498
                  tunnel: w497 -> [w507]
                  tunnel: [w506] -> w493
                  tunnel: w492 -> [w506]
                  tunnel: [w505] -> w488
                  tunnel: w487 -> [w505]
                  tunnel: [w504] -> w485
                  tunnel: w484 -> [w504]
                  tunnel: w483 -> [w503]
                  tunnel: [w502] -> w480
                  tunnel: w479 -> [w502]
                  tunnel: [w501] -> w473
                  tunnel: w472 -> [w501]
                  tunnel: [w516] -> w500
                  tunnel: w498 -> [w515]
                  tunnel: [w514] -> w494
                  tunnel: w493 -> [w514]
                  tunnel: [w513] -> w489
                  tunnel: w488 -> [w513]
                  tunnel: [w512] -> w486
                  tunnel: w485 -> [w512]
                  tunnel: [w511] -> w481
                  tunnel: w480 -> [w511]
                  tunnel: [w510] -> w474
                  tunnel: w473 -> [w510]
                  tunnel: w500 -> [w524]
                  tunnel: [w524] -> w499
                  tunnel: [w523] -> w495
                  tunnel: w494 -> [w523]
                  tunnel: w489 -> [w522]
                  tunnel: w486 -> [w521]
                  tunnel: [w520] -> w482
                  tunnel: w481 -> [w520]
                  tunnel: [w517] -> w478
                  tunnel: [w518] -> w477
                  tunnel: [w519] -> w475
                  tunnel: w474 -> [w519]
                  tunnel: [w518] -> w471
                  tunnel: [w517] -> w470
                  tunnel: [w537] -> w496
                  tunnel: w499 -> [w537]
                  tunnel: [w536] -> w491
                  tunnel: w495 -> [w536]
                  tunnel: w482 -> [w534]
                  tunnel: w478 -> [w528]
                  tunnel: w477 -> [w529]
                  tunnel: [w532] -> w476
                  tunnel: w475 -> [w531]
                  tunnel: w471 -> [w527]
                  tunnel: w470 -> [w526]
                  frame #0 {
                    n125 = Multiply(x=w503, y=1000.0) -> (x*y=w509:dbl)
                    n126 = Wait (ms)(milliseconds to wait=w509) -> ()  [unwired: 1 out]
                  }
                  frame #1 {
                    n127 = call <vilib>:"Wait at Rendezvous.vi"("rendezvous"=w515) -> ("error out"=w516:errorcluster)  [unwired: 4 in, 2 out]
                  }
                  frame #2 {
                    n128 = call "ReadSpectrum(SubVI).vi"("Continuous \nStrobe Delay"=w521, "Enter the \nInetegration Time"=w522) -> ("Spectrum Values"=w517:dbl[], "WL Values"=w518:dbl[], "Number of Spectrometers"=w525:i32)  [unwired: 7 in]
                    n129 = property on="Number of Spectrometers" class="DigNum (strict)"("Value"=w525) -> ()  [unwired: 2 in, 2 out]
                  }
                  frame #3 {
                    n130 = Equal?(x=1, y=w534) -> (x = y?=w535:bool)
                    n131 = case shown="False" w535 {
                      tunnel: [w538 w544] -> w532
                      tunnel: w527 -> [w539 w542]
                      tunnel: w526 -> [_ w541]
                      tunnel: w531 -> [w540 w543]
                      frame False {
                        # "Intensity thereafter"
                        n132 = Build Array (concatenate)(w540, w539) -> (w538:dbl[][])
                      }
                      frame True {
                        # "WL + Int on first iteration"
                        n133 = Build Array (concatenate)(w543, w542, w541) -> (w544:dbl[][])
                      }
                    }
                    n134 = Bundle("WL Values"=w529, "Spectrum Values"=w528) -> (→"?":T1)  [unwired: 1 in]
                  }
                }
                n135 = Wait on Notification(notifier=w491) -> (notification=w490:bool)  [unwired: 3 in, 3 out]
              }
              n136 = while {
                tunnel: w435 -> [w451]
                tunnel: w431 -> [w450]
                tunnel: [w448] -> w432
                shift-right: [w441] -> w425
                shift-left: w422 -> [w444]
                tunnel: [w439] -> w426
                stop <- w449 stop-if-true
                n137 = flat-sequence {
                  tunnel: w451 -> [w460]
                  tunnel: w444 -> [w465]
                  tunnel: [w463] -> w443
                  tunnel: w443 -> [w469]
                  tunnel: [w466] -> w439
                  frame #0 {
                    n138 = call <vilib>:"Wait at Rendezvous.vi"("rendezvous"=w460) -> ()  [unwired: 4 in, 3 out]
                  }
                  frame #1 {
                    n139 = Unbundle By Name(w465) -> ("Start time"=w461:i32)
                    n140 = Tick Count (ms)() -> (millisecond timer value=w462:u32)
                    n141 = Subtract(x=w462, y=w461) -> (x-y=w464:u32)
                    n142 = Bundle By Name(cluster=w465, "Time elapsed"=w464) -> (w463:T8)
                  }
                  frame #2 {
                    n143 = local read "V (during measurment)"() -> (w467:dbl)
                    n144 = Unbundle By Name(w469) -> ("V 1"=w468:dbl)
                    n145 = Equal?(x=w468, y=w467) -> (x = y?=w466:bool)
                  }
                }
                n146 = case shown="False" w439 {
                  tunnel: w443 -> [w455 w459]
                  tunnel: [w452 w458] -> w449
                  tunnel: [w454 w456] -> w440
                  tunnel: [w453 w457] -> w446
                  frame False {
                    n147 = Unbundle By Name(w455) -> ("Time elapsed"=w454:i32, "V 2"=w453:dbl)
                    n148 = Greater Or Equal?(x=w454, y=w453) -> (x >= y?=w452:bool)
                  }
                  frame True {
                    n149 = Unbundle By Name(w459) -> ("Time elapsed"=w456:i32, "V1 time"=w457:dbl)
                    n150 = Greater Or Equal?(x=w456, y=w457) -> (x >= y?=w458:bool)
                  }
                }
                n151 = Unbundle By Name(w443) -> ("Time array"=w447:dbl[])
                n152 = Coerce To Type(0:w440, 1:w446) -> (2:w445:dbl)
                n153 = Send Notification(notification=w449, notifier=w450) -> (notifier out=w448:refnum<notifier>)  [unwired: 1 in, 1 out]
                n154 = Build Array (concatenate)(w447, w445) -> (w442:dbl[])
                n155 = Bundle By Name(cluster=w443, "Time array"=w442) -> (w441:T8)
              }
              n156 = while {
                shift-right: [w559] -> w418
                shift-left: w417 -> [w558]
                tunnel: w435 -> [w556]
                tunnel: w431 -> [w553]
                shift-right: [w550] -> w420
                shift-left: w421 -> [w545]
                stop <- w551 stop-if-true
                n157 = flat-sequence {
                  tunnel: [w566] -> w561
                  tunnel: w558 -> [w565]
                  tunnel: [w564] -> w557
                  tunnel: w556 -> [w564]
                  tunnel: [w563] -> w554
                  tunnel: w553 -> [w563]
                  tunnel: [w562] -> w546
                  tunnel: w545 -> [w562]
                  tunnel: [w572] -> w560
                  tunnel: w561 -> [w573]
                  tunnel: w557 -> [w571]
                  tunnel: [w570] -> w555
                  tunnel: w554 -> [w570]
                  tunnel: [w569] -> w547
                  tunnel: w546 -> [w569]
                  tunnel: [w578] -> w559
                  tunnel: [w574] -> w549
                  tunnel: w560 -> [w577]
                  tunnel: [w576] -> w552
                  tunnel: w555 -> [w576]
                  tunnel: [w575] -> w548
                  tunnel: w547 -> [w575]
                  frame #0 {
                    n158 = call "IV getcurrent.vi"("error in (no error)"=w565) -> ("error out"=w566:errorcluster, "value out"=w568:dbl)  [unwired: 8 in, 1 out]
                    n159 = call "Current ranging routine (SubVI).vi"("Current"=w568) -> ()  [unwired: 11 in]
                    n160 = Wait (ms)(milliseconds to wait=u32 100) -> ()  [unwired: 1 out]
                  }
                  frame #1 {
                    n161 = call <vilib>:"Wait at Rendezvous.vi"("error in (no error)"=w573, "rendezvous"=w571) -> ("error out"=w572:errorcluster)  [unwired: 3 in, 2 out]
                  }
                  frame #2 {
                    # "Building a 1d matrix of currents"
                    n162 = call "IV getcurrent.vi"("error in (no error)"=w577) -> ("error out"=w578:errorcluster, "value out"=w574:dbl)  [unwired: 8 in, 1 out]
                    "System potential" <- w574
                  }
                }
                n163 = Build Array (concatenate)(w548, w549) -> (w550:dbl[])
                n164 = Wait on Notification(notifier=w552) -> (notification=w551:bool)  [unwired: 3 in, 3 out]
              }
              n165 = case shown="False" w426 {
                tunnel: [OSSPEC."Reinitialise Cell" OSSPEC."Apply V2"] -> w424
                frame False {
                }
                frame True {
                }
              }
              n166 = Release Notifier(notifier=w432) -> ()  [unwired: 2 in, 3 out]
              n167 = Merge Errors(w416, w418) -> (w419:errorcluster)
            }
            frame "Reinitialise Cell" {
              n168 = flat-sequence {
                tunnel: w588 -> [w591]
                tunnel: [w590] -> w586
                tunnel: [w594] -> w587
                tunnel: w586 -> [w594]
                tunnel: w587 -> [w598]
                tunnel: [w597] -> w585
                frame #0 {
                  # "off"
                  n169 = To Long Integer(number=0) -> (32bit integer=w593:i32)
                  n170 = local write "cell on"(FALSE ("cell on")) -> ()
                  n171 = call "IV setcellon.vi"("error in (no error)"=w591, "cellon"=w593) -> ("error out"=w590:errorcluster)  [unwired: 7 in, 2 out]
                }
                frame #1 {
                  n172 = Wait (ms)(milliseconds to wait=u32 100) -> ()  [unwired: 1 out]
                }
                frame #2 {
                  # "on"
                  n173 = local write "cell on"(TRUE ("cell on")) -> ()
                  n174 = To Long Integer(number=1) -> (32bit integer=w600:i32)
                  n175 = call "IV setcellon.vi"("error in (no error)"=w598, "cellon"=w600) -> ("error out"=w597:errorcluster)  [unwired: 7 in, 2 out]
                }
              }
              n176 = Unbundle By Name(w582) -> ("Spectrum"=w581:dbl[][], "Current array"=w580:dbl[], "Potential array"=w579:dbl[])
            }
            frame "Apply V1" {
              n177 = flat-sequence {
                tunnel: w613 -> [w617]
                tunnel: [w618] -> w614
                tunnel: w607 -> [w615]
                tunnel: w614 -> [w633]
                tunnel: w613 -> [w631]
                tunnel: [w632] -> w612
                tunnel: [w630] -> w610
                tunnel: w612 -> [w636]
                tunnel: [w636] -> w611
                tunnel: w610 -> [w635]
                tunnel: [w635] -> w609
                tunnel: w611 -> [w639]
                tunnel: w609 -> [w637]
                tunnel: [w638] -> w608
                tunnel: [w637] -> w604
                frame #0 {
                  n178 = Unbundle By Name(w617) -> ("V 1"=w616:dbl)
                  n179 = Absolute Value(x=w616) -> (abs(x)=w621:dbl)
                  n180 = Greater?(x=w621, y=3.0) -> (0:w619:bool)
                  n181 = case shown="True" w619 {
                    tunnel: [w622 w624] -> w618
                    tunnel: w615 -> [w622 w623]
                    frame False {
                    }
                    frame True {
                      # "abort if E >3 V"
                      n182 = call "IV setcellon.vi"("error in (no error)"=w623, "cellon"=0) -> ("error out"=w626:errorcluster)  [unwired: 7 in, 2 out]
                      n183 = call "IV close.vi"("error in (no error)"=w626) -> ("error out"=w624:errorcluster)  [unwired: 9 in, 1 out]
                      n184 = call "Display Message to User3"("error in (no error)"=w624) -> ("OK"=w627:bool)  [unwired: 9 in, 1 out]
                      n185 = Stop(stop? (T)=w627) -> ()
                    }
                  }
                  n186 = local write "V (during measurment)"(w616) -> ()
                }
                frame #1 {
                  n187 = Tick Count (ms)() -> (millisecond timer value=w629:u32)
                  n188 = call "IV setpotential.vi"("error in (no error)"=w633) -> ("error out"=w632:errorcluster)  [unwired: 8 in, 2 out]
                  n189 = Bundle By Name(cluster=w631, "Start time"=w629, "Time elapsed"=0) -> (w630:T8)
                }
                frame #2 {
                  n190 = Wait (ms)(milliseconds to wait=u32 100) -> ()  [unwired: 1 out]
                }
                frame #3 {
                  n191 = call "IV getcurrent.vi"("error in (no error)"=w639) -> ("error out"=w638:errorcluster, "value out"=w640:dbl)  [unwired: 8 in, 1 out]
                  n192 = call "Current ranging routine (SubVI).vi"("Current"=w640) -> ()  [unwired: 11 in]
                }
              }
              n193 = Unbundle By Name(w604) -> ("Spectrum"=w603:dbl[][], "Current array"=w602:dbl[], "Potential array"=w601:dbl[])
            }
            frame "Apply V2" {
              n194 = flat-sequence {
                tunnel: w644 -> [w654]
                tunnel: [w655] -> w651
                tunnel: w647 -> [w653]
                tunnel: w651 -> [w666]
                tunnel: [w665] -> w650
                tunnel: w650 -> [w668]
                tunnel: [w668] -> w649
                tunnel: w649 -> [w670]
                tunnel: [w669] -> w648
                frame #0 {
                  n195 = Unbundle By Name(w654) -> ("V 2"=w652:dbl)
                  n196 = Absolute Value(x=w652) -> (abs(x)=w658:dbl)
                  n197 = Greater?(x=w658, y=3.0) -> (0:w656:bool)
                  n198 = case shown="True" w656 {
                    tunnel: [w659 w661] -> w655
                    tunnel: w653 -> [w659 w660]
                    frame False {
                    }
                    frame True {
                      # "abort if E >3 V"
                      n199 = call "IV setcellon.vi"("error in (no error)"=w660, "cellon"=0) -> ("error out"=w663:errorcluster)  [unwired: 7 in, 2 out]
                      n200 = call "IV close.vi"("error in (no error)"=w663) -> ("error out"=w661:errorcluster)  [unwired: 9 in, 1 out]
                      n201 = call "Display Message to User4"("error in (no error)"=w661) -> ("OK"=w664:bool)  [unwired: 9 in, 1 out]
                      n202 = Stop(stop? (T)=w664) -> ()
                    }
                  }
                  n203 = local write "V (during measurment)"(w652) -> ()
                }
                frame #1 {
                  n204 = call "IV setpotential.vi"("error in (no error)"=w666) -> ("error out"=w665:errorcluster)  [unwired: 8 in, 2 out]
                }
                frame #2 {
                  n205 = Wait (ms)(milliseconds to wait=u32 100) -> ()  [unwired: 1 out]
                }
                frame #3 {
                  n206 = call "IV getcurrent.vi"("error in (no error)"=w670) -> ("error out"=w669:errorcluster, "value out"=w671:dbl)  [unwired: 8 in, 1 out]
                  n207 = call "Current ranging routine (SubVI).vi"("Current"=w671) -> ()  [unwired: 11 in]
                }
              }
              n208 = Unbundle By Name(w644) -> ("Spectrum"=w643:dbl[][], "Current array"=w642:dbl[], "Potential array"=w641:dbl[])
            }
          }
          n209 = Bundle By Name(cluster=w288, "Spectrum"=w287, "Current array"=w286, "Potential array"=w284) -> (w285:T8)
        }
      }
      frame "Output data and process" {
        # "Also re-intialise constants"
      }
    }
    n210 = Equal To 0?(x=w21) -> (x = 0?=w32:bool)
    n211 = case shown="False" w32 {
      tunnel: w33 -> [w51 w77]
      tunnel: [w50 w75] -> w25
      tunnel: [w45 w69] -> w31
      tunnel: [w46 w70] -> w18
      tunnel: [w48 w76] -> w19
      tunnel: [w44 w68] -> w23
      tunnel: [w47 w71] -> w24
      frame False {
        n212 = call "IV getcellstatus.vi"() -> ("devcellstatus out"=w61:i32)  [unwired: 9 in, 2 out]
        n213 = call "Bitget 8-bits test.vi"("x"=w61) -> ("c"=w57:dbl, "e"=w59:dbl, "f"=w58:dbl, "h"=w60:dbl)  [unwired: 19 in, 4 out]
        n214 = Greater?(x=w57, y=0.0) -> (0:w63:bool)
        n215 = Greater?(x=w59, y=0.0) -> (0:w64:bool)
        n216 = Greater?(x=w58, y=0.0) -> (0:w65:bool)
        n217 = Greater?(x=w60, y=0.0) -> (0:w43:bool)
        n218 = And(x=w61, y=256) -> (x .and. y?=w62:i32)
        n219 = Equal?(x=w62, y=256) -> (x = y?=w66:bool)
        n220 = Bundle By Name(cluster=w51, "I overload"=w63, "Aninput1 overload"=w64, "E overload"=w65, "Cell of button pressed"=w43, "Cell on"=w66) -> (w50:T8)
        n221 = Unbundle By Name(w50) -> ("I overload"=w48:bool, "Aninput1 overload"=w47:bool, "E overload"=w46:bool, "Cell of button pressed"=w45:bool, "Cell on"=w44:bool)
      }
      frame True {
        w67 = FALSE
        # "After closing the driver reset the indicators"
        n222 = property class="XYGraph (strict)"("Value"=cluster{dbl[], dbl[]} {[], []} ("XY Graph")) -> ()  [unwired: 2 in, 2 out]
        n223 = property on="Potentiostat Status" class="Str"("Value"="" ("Device Status indicator")) -> ()  [unwired: 2 in, 2 out]
        n224 = property on="Device serial number" class="Str"("Value"="" ("Device serial number")) -> ()  [unwired: 2 in, 2 out]
        n225 = Bundle By Name(cluster=w77, "I overload"=w67, "Aninput1 overload"=w67, "E overload"=w67, "Cell of button pressed"=w67, "Cell on"=w67) -> (w75:T8)
        n226 = Unbundle By Name(w75) -> ("I overload"=w76:bool, "Aninput1 overload"=w71:bool, "E overload"=w70:bool, "Cell of button pressed"=w69:bool, "Cell on"=w68:bool)
      }
    }
    "I_overload" <- w19
    "Aninput1_overload" <- w24
    "E_overload" <- w18
    "cell-off button pressed" <- w31
    "cell on" <- w23
    n227 = Unbundle By Name(w33) -> ("Current"=→"current":dbl, "Serial No"=→"Device serial number":string, "Status"=→"Potentiostat Status":string)
    n228 = Or(x=w26, y=w38) -> (x .or. y?=w37:bool)
    n229 = Or(x=w19, y=w18) -> (x .or. y?=w17:bool)
    n230 = case shown="True" w17 {
      tunnel: w16 -> [w41 _]
      tunnel: [w41 State."Exit" ("f")] -> w20
      frame False {
      }
      frame True {
        n231 = call "Display Message to User"() -> ()  [unwired: 10 in, 2 out]
      }
    }
  }
